vi "Read Channel List.vi"(8 "error in":errorcluster, 11 "ChanMngOOB_Tx in":refnum<class "ChnMngOOB_Tx.lvclass">) -> (0 "error out":errorcluster, 2 "Channel List":T1[](array[typedef]), 3 "ChanMngOOB_Tx out":refnum<class "ChnMngOOB_Tx.lvclass">)   [LabVIEW 2021, in "ChnMngOOB_Tx.lvclass"]
uses:
  ChnMngOOB_Tx.lvclass
  C:/Program Files/National Instruments/LabVIEW 2021/vi.lib/CIF Foundation/CIF Out of Band Commands/CIFOutOfBand.lvclass
  typedef/Channel List for OOB.ctl
  <vilib>/CIF Foundation/CIF Channels Core/CIFChannels/Typedef/Direction.ctl
  <vilib>/CIF Foundation/CIF Out of Band Commands/CIFOutOfBand.lvclass/CIFOutOfBand.ctl
  <vilib>/CIF Foundation/CIF Out of Band Commands/Accessors/Read Local OOB Data.vi
  <vilib>/CIF Foundation/CIF Channels Core/CIFChannels/CIFChannels.lvclass
  CIFChannelMng.lvclass
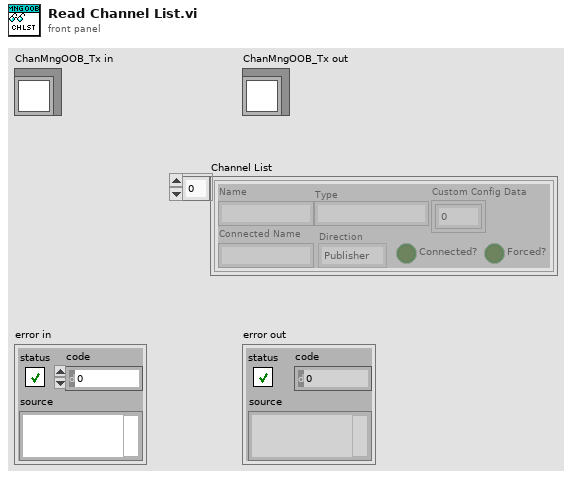
[diagram p1: front panel]
types:
  T1 = typedef "CIFChannelMng.lvclass/Channel List for OOB.ctl" = cluster{"Name":string, "Direction":T2, "Type":string, "Connected?":bool, "Connected Name":string, "Custom Config Data":u8[], "Forced?":bool}
  T2 = typedef "CIFChannels.lvclass/Direction.ctl" = enum16{"Publisher", "Subscriber"}
  T3 = typedef "ChnMngOOB_Tx.lvclass/Template Payload.ctl" = cluster{"Channel List":T1[], "New FIFO Publisher":T4}
  T4 = typedef "ChnMngOOB_Tx.lvclass/FIFO Publisher Return.ctl" = cluster{"FIFO Pub Name":string, "error":errorcluster, "Added":bool}
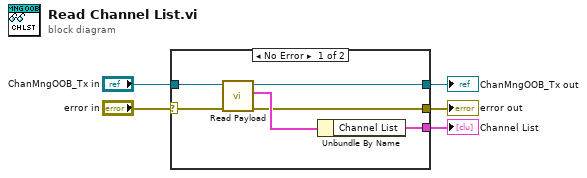
[diagram p0: block diagram]
diagram:
  n1 = case shown="No Error" "error in" {
    selector: "error in" -> [w7 w12]
    tunnel: [w6 w12] -> w4
    tunnel: [w10 w13] -> w2
    tunnel: "ChanMngOOB_Tx in" -> [w11 w13]
    tunnel: [w8 _] -> w1
    frame No Error {
      n2 = call "Read Payload.vi"("error in"=w7, "ChanMngOOB_Tx in"=w11) -> ("error out"=w6:errorcluster, "data"=w9:T3, "ChanMngOOB_Tx out"=w10:refnum<class "ChnMngOOB_Tx.lvclass">)  [unwired: 7 in]
      n3 = Unbundle By Name(w9) -> ("Channel List"=w8:T1[])
    }
    frame Error {
    }
  }
  "error out" <- w4
  "ChanMngOOB_Tx out" <- w2
  "Channel List" <- w1
